vi "INST_PS_SET_VOLTAGE_LEVEL_4.0.0.vi"(4 "Use OPC(T)":bool, 6 "Instrument Select (Output 1)":string(combo), 7 "SEL_PS":string(combo), 8 "error in (no error)":errorcluster, 9 "Voltage (0.0)":dbl format="%.2p", 10 "Voltage (0.0)str":string, 11 "VISA session":refnum<visa-resource-name>) -> (0 "error out":errorcluster, 3 "dup VISA session":refnum<visa-resource-name>)   [LabVIEW 2018]
doc: "This VI configures the DC voltage level the power supply attempts to generate.\n\nVer 3.0.0 supports the E36xx Model and The 6634B based on the GPIB address of idtATE [10-12]"
uses:
  Initialize References/Station References Global.vi
panel:
  out "PSn Model":string
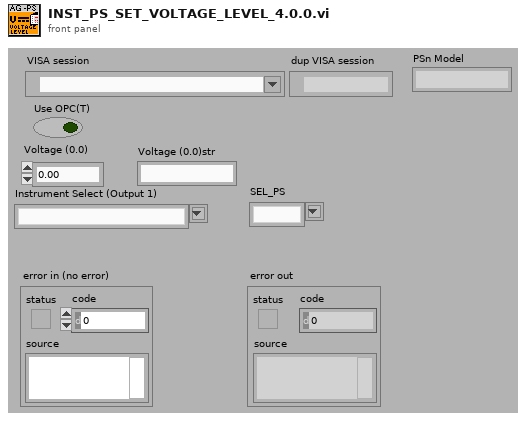
[diagram p1: front panel]
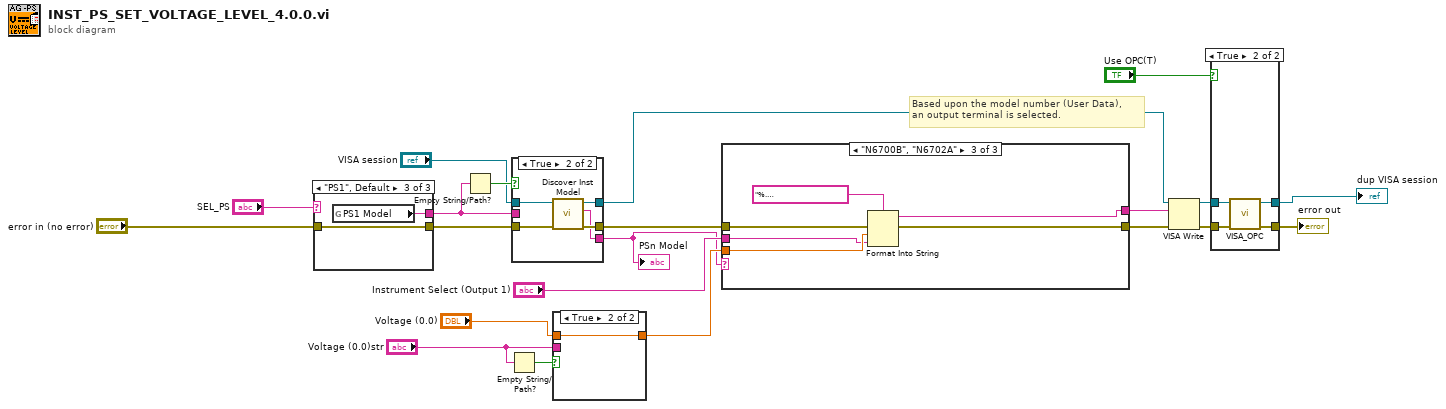
[diagram p0: block diagram]
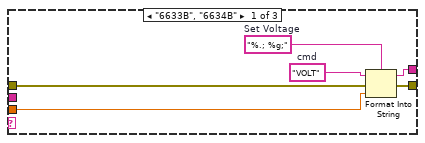
[diagram p2: hidden frame]
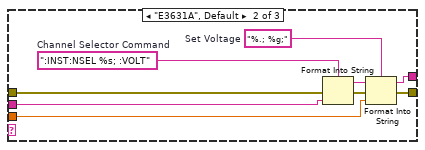
[diagram p3: hidden frame]
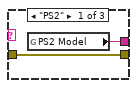
[diagram p5: hidden frame]
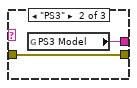
[diagram p6: hidden frame]
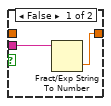
[diagram p7: hidden frame]
diagram:
  # "Based upon the model number (User Data), \nan output terminal is selected."
  n1 = case shown="\"PS1\", Default" "SEL_PS" {
    tunnel: [w23 w25 w27] -> w1
    tunnel: "error in (no error)" -> [w22 w24 w26]
    tunnel: [w22 w24 w26] -> w4
    frame "PS2" {
      n2 = global read "Station References Global.vi" "PS2 Model"() -> (w23:string)
    }
    frame "PS3" {
      n3 = global read "Station References Global.vi" "PS3 Model"() -> (w25:string)
    }
    frame "PS1", Default {
      n4 = global read "Station References Global.vi" "PS1 Model"() -> (w27:string)
    }
  }
  n5 = Empty String/Path?(string/path=w1) -> (empty?=w7:bool)
  n6 = Empty String/Path?(string/path="Voltage (0.0)str") -> (empty?=w14:bool)
  n7 = case shown="True" w7 {
    tunnel: "VISA session" -> [w30 w35]
    tunnel: [w30 w34] -> w5
    tunnel: w4 -> [w28 w33]
    tunnel: [w28 w32] -> w3
    tunnel: [w29 w31] -> w2
    tunnel: w1 -> [w29 _]
    frame False {
    }
    frame True {
      n8 = call "Discover Inst Model.vi"("error in"=w33, "Session In"=w35) -> ("error out"=w32:errorcluster, "Model #"=w31:string, "Session Out"=w34:refnum<visa-resource-name>)  [unwired: 7 in]
    }
  }
  "PSn Model" <- w2
  n9 = case shown="True" w14 {
    tunnel: "Voltage (0.0)str" -> [w37 _]
    tunnel: [w36 w38] -> w13
    tunnel: "Voltage (0.0)" -> [_ w38]
    frame False {
      n10 = Fract/Exp String To Number(string=w37) -> (number=w36:dbl)  [unwired: 3 in, 1 out]
    }
    frame True {
    }
  }
  n11 = case shown="\"N6700B\", \"N6702A\"" w2 {
    tunnel: w13 -> [w41 w50 w58]
    tunnel: "Instrument Select (Output 1)" -> [_ w49 w56]
    tunnel: [w43 w48 w57] -> w11
    tunnel: w3 -> [w40 w47 w55]
    tunnel: [w39 w45 w54] -> w8
    frame "6633B", "6634B" {
      w42 = "VOLT"  # cmd
      w44 = "%.; %g;"  # Set Voltage
      n12 = Format Into String(format string=w44, initial string=w42, error in=w40, w41) -> (resulting string=w43:string, error out=w39:errorcluster)
    }
    frame "E3631A", Default {
      w51 = ":INST:NSEL %s; :VOLT"  # Channel Selector Command
      w53 = "%.; %g;"  # Set Voltage
      n13 = Format Into String(format string=w51, error in=w47, w49) -> (resulting string=w52:string, error out=w46:errorcluster)  [unwired: 1 in]
      n14 = Format Into String(format string=w53, initial string=w52, error in=w46, w50) -> (resulting string=w48:string, error out=w45:errorcluster)
    }
    frame "N6700B", "N6702A" {
      n15 = Format Into String(format string="%.;SOUR:VOLT:LEV:IMM:AMPL %.;%Le,(@%s)", error in=w55, w58, w56) -> (resulting string=w57:string, error out=w54:errorcluster)  [unwired: 1 in]
    }
  }
  n16 = VISA Write(VISA resource name=w5, write buffer=w11, error in (no error)=w8) -> (VISA resource name out=w21:refnum<visa-resource-name>, error out=w20:errorcluster)  [unwired: 1 out]
  n17 = case shown="True" "Use OPC(T)" {
    tunnel: w20 -> [w61 w64]
    tunnel: [w61 w65] -> w17
    tunnel: w21 -> [w60 w63]
    tunnel: [w60 w62] -> w18
    frame False {
    }
    frame True {
      n18 = call "VISA_OPC.vi"("error in"=w64, "Session In"=w63) -> ("error out"=w65:errorcluster, "Session Out"=w62:refnum<visa-resource-name>)  [unwired: 7 in, 1 out]
    }
  }
  "error out" <- w17
  "dup VISA session" <- w18
